vi "Math result Sorting.vi"(6 "sort method":enum16{"sort by x axis", "sort by y axis"}(ring), 8 "error in":errorcluster, 10 "Matches (pixel)":T1(array[cluster])) -> (0 "error out":errorcluster, 2 "Matches (pixel)":T1(array[cluster]))   [LabVIEW 2017]
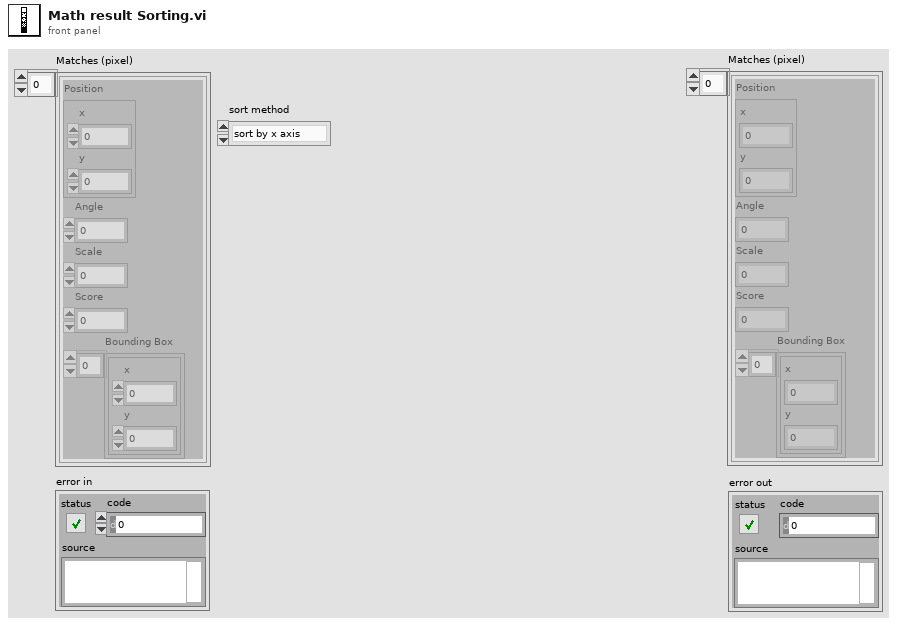
[diagram p1: front panel]
types:
  T1 = cluster{"Position":cluster{"x":sgl, "y":sgl}, "Angle":sgl, "Scale":sgl, "Score":sgl, "Bounding Box":cluster{"x":sgl, "y":sgl}[]}[]
  T2 = cluster{"Position":cluster{"x":sgl, "y":sgl}, "Angle":sgl, "Scale":sgl, "Score":sgl, "Bounding Box":cluster{"x":sgl, "y":sgl}[]}
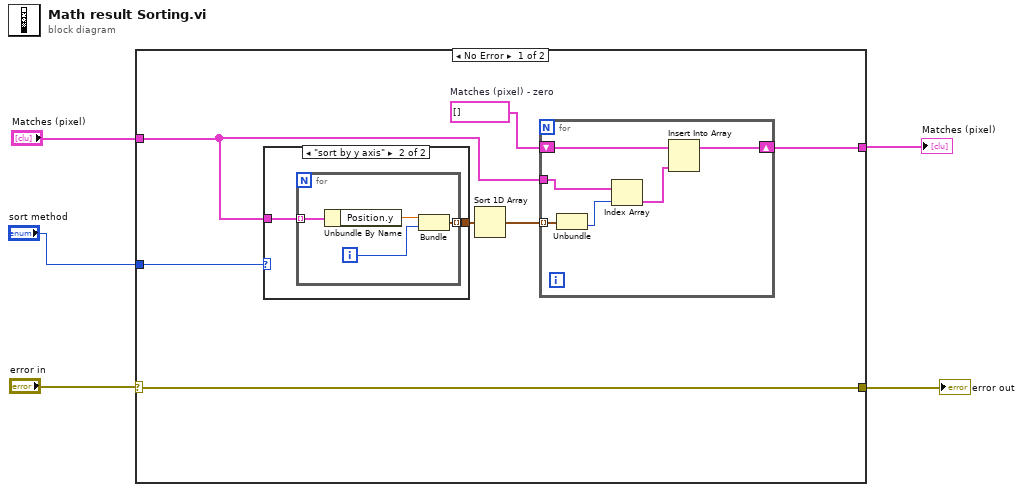
[diagram p0: block diagram]
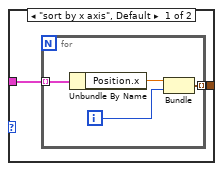
[diagram p2: hidden frame]
diagram:
  n1 = case shown="No Error" "error in" {
    selector: "error in" -> [w12 w32]
    tunnel: [w12 w32] -> w4
    tunnel: "Matches (pixel)" -> [w10 w31]
    tunnel: [w7 w31] -> w2
    tunnel: "sort method" -> [w6 _]
    frame No Error {
      w9 = T1 []  # Matches (pixel) - zero
      n2 = case shown="\"sort by y axis\"" w6 {
        tunnel: [w14 w20] -> w11
        tunnel: w10 -> [w13 w19]
        frame "sort by x axis", Default {
          n3 = for {
            tunnel: w13 -> [w18] mode=indexing
            tunnel: [w15] -> w14 mode=indexing
            i -> [w16]
            n4 = Unbundle By Name(w18) -> ("Position.x"=w17:sgl)
            n5 = Bundle("x"=w17, w16) -> (w15:cluster{"x":sgl, i32})  [unwired: 1 in]
          }
        }
        frame "sort by y axis" {
          n6 = for {
            tunnel: w19 -> [w24] mode=indexing
            tunnel: [w21] -> w20 mode=indexing
            i -> [w22]
            n7 = Unbundle By Name(w24) -> ("Position.y"=w23:sgl)
            n8 = Bundle("y"=w23, w22) -> (w21:cluster{"y":sgl, i32})  [unwired: 1 in]
          }
        }
      }
      n9 = Sort 1D Array(array=w11) -> (sorted array=w8:cluster{"y":sgl, i32}[])
      n10 = for {
        tunnel: w10 -> [w29]
        shift-right: [w26] -> w7
        shift-left: w9 -> [w27]
        tunnel: w8 -> [w30] mode=indexing
        n11 = Unbundle(w30) -> (w28:i32)  [unwired: 1 out]
        n12 = Index Array(array=w29, index=w28) -> (element=w25:T2)
        n13 = Insert Into Array(array=w27, new element=w25) -> (w26:T1)  [unwired: 1 in]
      }
    }
    frame Error {
    }
  }
  "error out" <- w4
  "Matches (pixel)" <- w2
